vi "Reading Delay.vi"(10 "Delay":u32=1000, 11 "In Range":bool) -> (3 "Take Reading":bool)   [LabVIEW 2013]
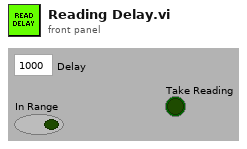
[diagram p1: front panel]
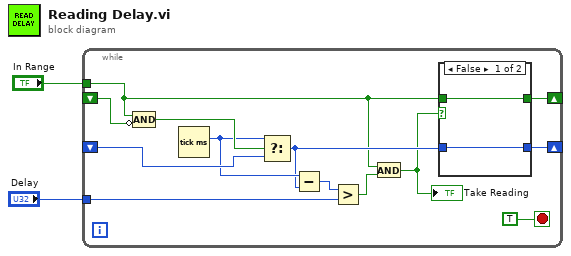
[diagram p0: block diagram]
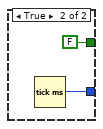
[diagram p2: hidden frame]
diagram:
  n1 = while {
    shift-right: [w4] -> _
    shift-left: _ -> [w10]
    shift-right: [w6] -> _
    shift-left: _ -> [w13]
    tunnel: "Delay" -> [w12]
    tunnel: "In Range" -> [w5]
    stop <- TRUE stop-if-true
    n2 = Compound Arithmetic op=AND(w5, invert w10) -> (w14:bool)
    n3 = Tick Count (ms)() -> (millisecond timer value=w9:u32)
    n4 = Select(t=w9, s=w14, f=w13) -> (s? t:f=w7:u32)
    n5 = Subtract(x=w9, y=w7) -> (x-y=w8:u32)
    n6 = Greater?(x=w8, y=w12) -> (0:w11:bool)
    n7 = And(x=w5, y=w11) -> (x .and. y?=w3:bool)
    "Take Reading" <- w3
    n8 = case shown="False" w3 {
      tunnel: [w17 w18] -> w6
      tunnel: w7 -> [w17 _]
      tunnel: [w16 FALSE ("In Range")] -> w4
      tunnel: w5 -> [w16 _]
      frame False {
      }
      frame True {
        n9 = Tick Count (ms)() -> (millisecond timer value=w18:u32)
      }
    }
  }
